vi "Get Dependencies.vi"(8 "error in (no error)":errorcluster, 11 "Instrument in":refnum<class "Instrument.lvclass">) -> (0 "error out":errorcluster, 2 "Dependencies":T1, 3 "SMO out":refnum<class "Instrument.lvclass">)   [LabVIEW 2016, in "Instrument.lvclass"]
uses:
  Instrument.lvclass
  RemoteControl/RemoteControl.lvclass
  Logger.DSC/Logger.DSC.lvclass
  Logger.Error/Logger.Error.lvclass
  C:/Program Files (x86)/National Instruments/LabVIEW 2016/vi.lib/JKI/JKI SMO/SMO/SMO.lvclass
  <vilib>/JKI/JKI SMO/SMO/SMO.lvclass
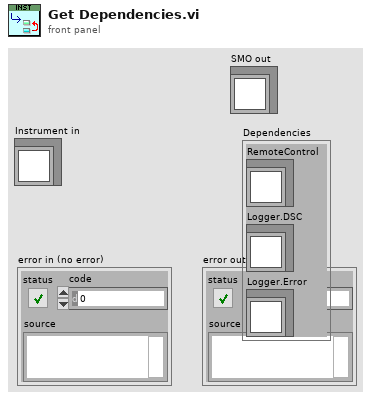
[diagram p1: front panel]
types:
  T1 = cluster{"RemoteControl":refnum<class "RemoteControl.lvclass">, "Logger.DSC":refnum<class "Logger.DSC.lvclass">, "Logger.Error":refnum<class "Logger.Error.lvclass">}
  T2 = cluster{"RemoteControl.lvclass":refnum<class "RemoteControl.lvclass">, "Logger.DSC.lvclass":refnum<class "Logger.DSC.lvclass">, "Logger.Error.lvclass":refnum<class "Logger.Error.lvclass">}
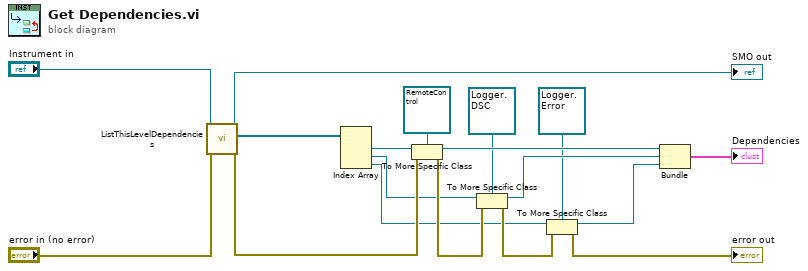
[diagram p0: block diagram]
diagram:
  n1 = call <vilib>:"ListThisLevelDependencies.vi"("error in (no error)"="error in (no error)", "SMO in"="Instrument in") -> ("error out"=w16:errorcluster, "[My Dependencies]"=w17:refnum<class "SMO.lvclass">[], "SMO out"=→"SMO out":refnum<class "Instrument.lvclass">)  [unwired: 7 in]
  n2 = Index Array(array=w17) -> (element #1=w18:refnum<class "SMO.lvclass">, element #2=w9:refnum<class "SMO.lvclass">, element #3=w3:refnum<class "SMO.lvclass">)  [unwired: 3 in]
  n3 = To More Specific Class(target class=refnum<class "RemoteControl.lvclass"> refnum ("RemoteControl.lvclass"), reference=w18, error in=w16) -> (specific class reference=w13:refnum<class "RemoteControl.lvclass">, error out=w15:errorcluster)
  n4 = To More Specific Class(target class=refnum<class "Logger.DSC.lvclass"> refnum ("Logger.DSC.lvclass"), reference=w9, error in=w15) -> (specific class reference=w12:refnum<class "Logger.DSC.lvclass">, error out=w8:errorcluster)
  n5 = To More Specific Class(target class=refnum<class "Logger.Error.lvclass"> refnum ("Logger.Error.lvclass"), reference=w3, error in=w8) -> (specific class reference=w4:refnum<class "Logger.Error.lvclass">, error out=→"error out":errorcluster)
  n6 = Bundle("RemoteControl.lvclass"=w13, "Logger.DSC.lvclass"=w12, "Logger.Error.lvclass"=w4) -> (→"Dependencies":T2)  [unwired: 1 in]
